vi "Module Loop.vi"(8 "error in (no error)":errorcluster, 11 "Config Alert Module in":refnum<class "Config Monitor Module.lvclass">) -> (0 "error out":errorcluster, 3 "Config Alert Module out":refnum<class "Config Monitor Module.lvclass">)   [LabVIEW 2020, in "Volatus.lvlib" / "Config Monitor Module.lvclass"]
uses:
  Config Monitor Module.lvclass
  C:/dev/lv20CE/relink/lv-volatus/Volatus/Module/Module.lvclass
  Node Config Info.ctl
  Module/Module.lvclass/Module.ctl
  MessageQ/MessageQ.lvclass/MessageQ.ctl
  Module/Module.lvclass
  Config Monitor Module.lvclass/Config Monitor Module.ctl
  ConfigMonitorInfoValue/ConfigMonitorInfoValue.lvclass/ConfigMonitorInfoValue.ctl
  Module/Parent Q.vi
  ConfigMonitorInfoValue/ConfigMonitorInfoValue.lvclass
  C:/dev/lv20CE/relink/lv-promises/Promises/Value/Value.lvclass
  <vilib>/Utility/error.llb/Error Cluster From Error Code.vi
  lv-promises/Promises/Promise/Promise.lvclass
  MessageQ/MessageQ.lvclass
panel:
  out "Config Hash":string
  out "Config Version":string
  in  "Array":T1[](array[typedef])
  # "This Node"
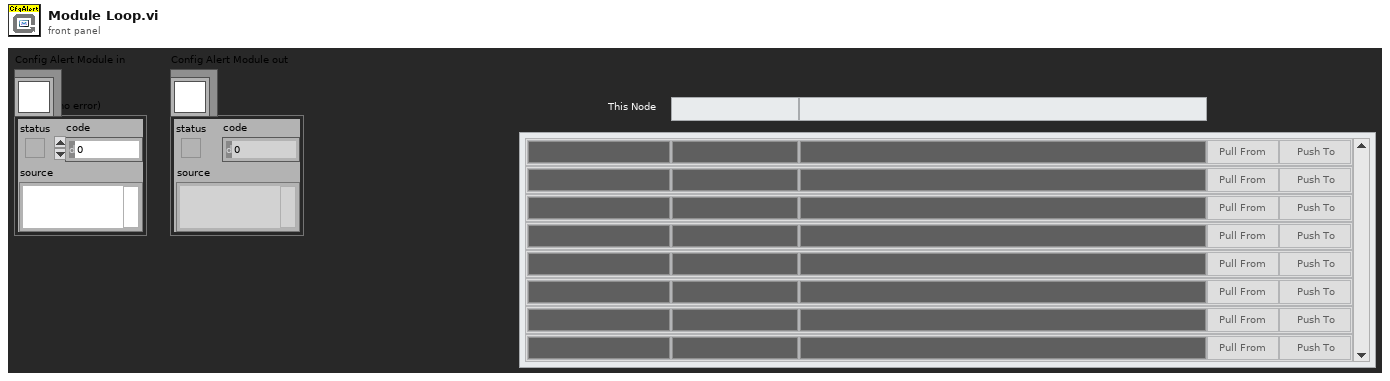
[diagram p1: front panel]
types:
  T1 = typedef "Volatus.lvlib/Config Monitor Module.lvclass/Node Config Info.ctl" = cluster{"Node":string, "Config Version":string, "Config Hash":string, "Pull":bool, "Push":bool, "Version Color":u32, "Hash Color":u32, "Node Color":u32}
  T2 = enum32{"Invalid", "Standard", "Closed", "Hidden", "Minimized", "Maximized"}
  T3 = cluster{"Node":bool, "Config Version":bool, "Config Hash":bool, "Pull":bool, "Push":bool, "Version Color":bool, "Hash Color":bool, "Node Color":bool}[]
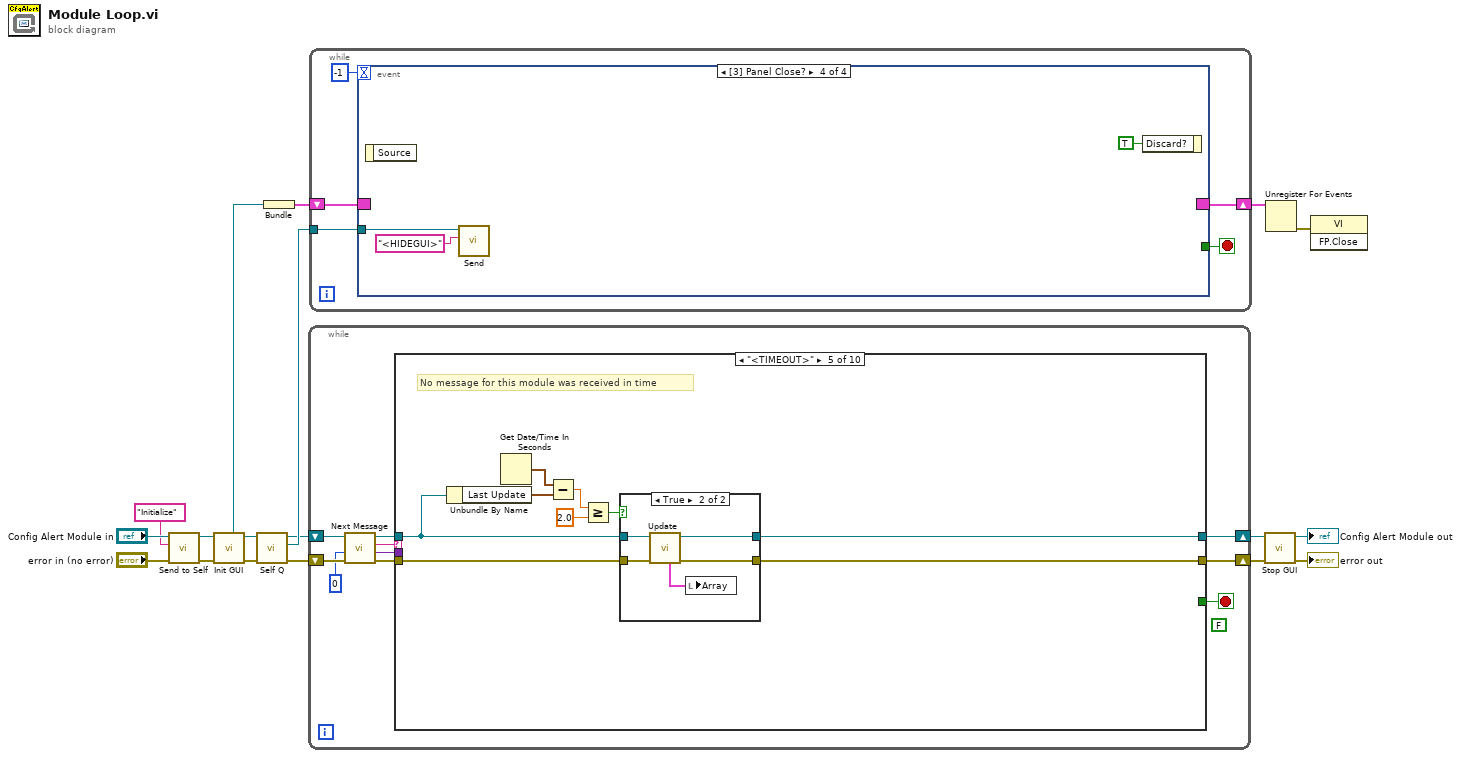
[diagram p0: block diagram]
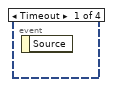
[diagram p2: hidden frame]
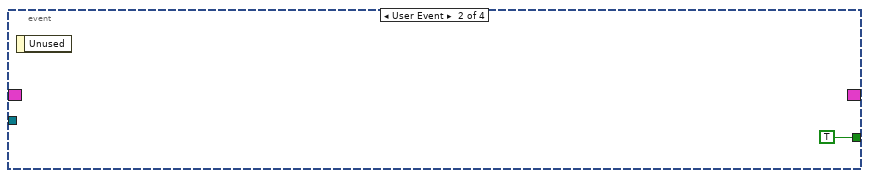
[diagram p3: hidden frame]
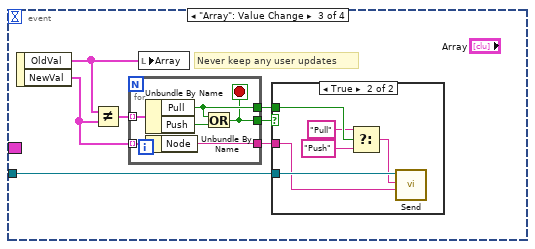
[diagram p4: hidden frame]
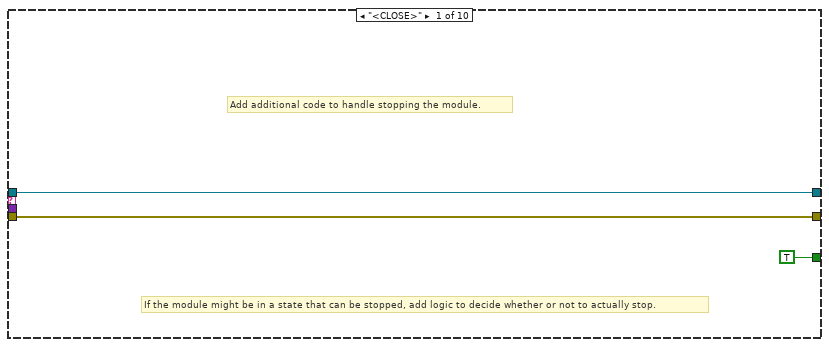
[diagram p6: hidden frame]
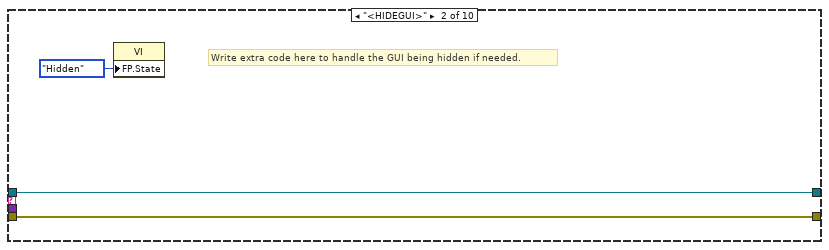
[diagram p7: hidden frame]
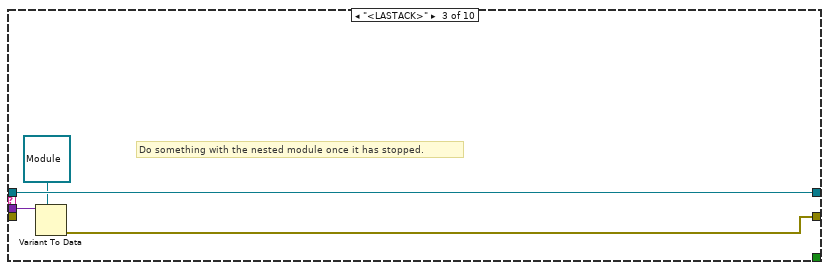
[diagram p8: hidden frame]
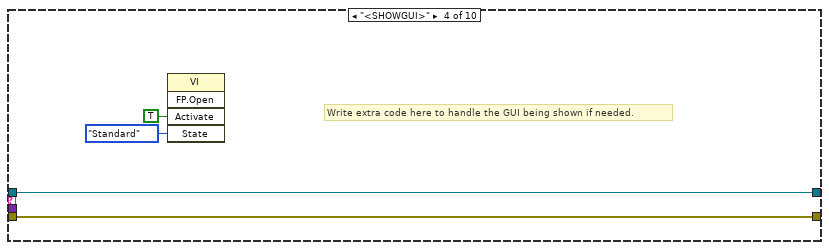
[diagram p9: hidden frame]
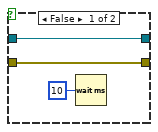
[diagram p10: hidden frame]
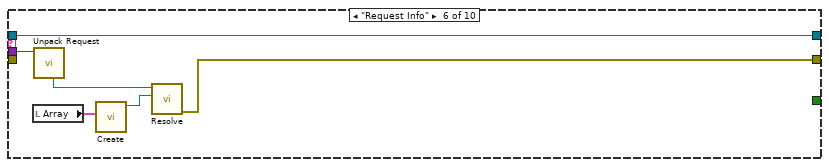
[diagram p11: hidden frame]
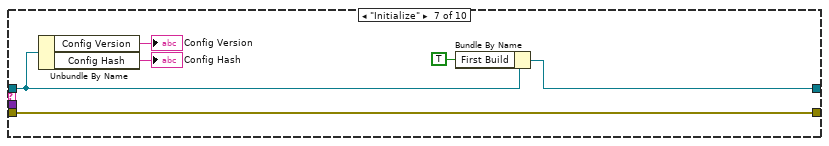
[diagram p12: hidden frame]
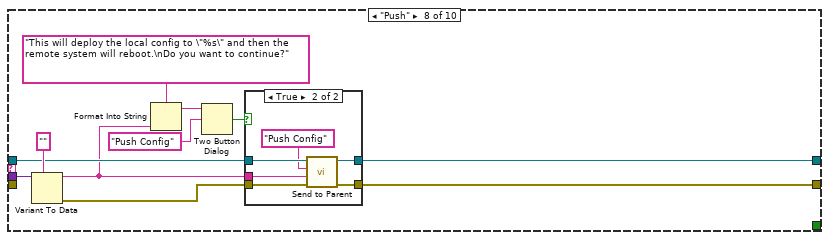
[diagram p13: hidden frame]
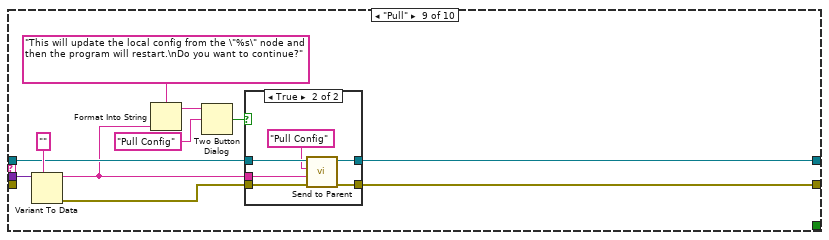
[diagram p15: hidden frame]
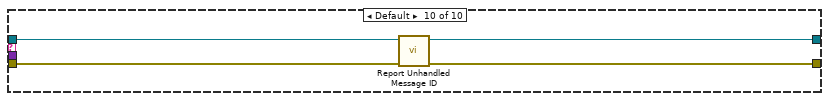
[diagram p17: hidden frame]
diagram:
  n1 = call "Send to Self.vi"("error in (no error)"="error in (no error)", "Message ID"="Initialize", "Module in"="Config Alert Module in") -> ("error out"=w4:errorcluster, "Module out"=w2:refnum<class "Config Monitor Module.lvclass">)  [unwired: 7 in]
  n2 = call "Init GUI.vi"("Module in"=w2) -> ("Module out"=w10:refnum<class "Config Monitor Module.lvclass">, "Event Reg"=w15:refnum<event-registration>)  [unwired: 9 in]
  n3 = call "Self Q.vi"("Module in"=w10) -> ("Self Q"=w9:refnum<class "MessageQ.lvclass">, "Module out"=w8:refnum<class "Config Monitor Module.lvclass">)  [unwired: 9 in]
  n4 = Bundle("Event Reg"=w15) -> (w11:cluster{"Event Reg":refnum<event-registration>})  [unwired: 1 in]
  n5 = while {
    shift-right: [w21] -> w13
    shift-left: w8 -> [w26]
    shift-right: [w20] -> w14
    shift-left: w4 -> [w25]
    stop <- w19 stop-if-true
    (unwired) FALSE
    n6 = call "Next Message.vi"("error in (no error)"=w25, "Timeout ms (-1)"=0, "Module in"=w26) -> ("error out"=w24:errorcluster, "Data"=w18:variant, "ID"=w23:string, "Module out"=w22:refnum<class "Config Monitor Module.lvclass">)  [unwired: 5 in]
    n7 = case shown="\"<TIMEOUT>\"" w23 {
      tunnel: w24 -> [w27 w31 _ w39 w49 _ w69 _ _ w111]
      tunnel: w22 -> [w28 w32 w36 w40 w46 w63 w68 w74 w93 w109]
      tunnel: [w28 w32 w36 w40 w47 w63 w65 w72 w91 w108] -> w21
      tunnel: [w27 w31 w33 w39 w48 w58 w69 w71 w90 w110] -> w20
      tunnel: [TRUE _ _ _ _ _ _ _ _ _] -> w19
      tunnel: w18 -> [_ _ w35 _ _ w62 _ w80 w99 _]
      frame "<CLOSE>" {
        # "If the module might be in a state that can be stopped, add logic to decide whether or not to actually stop."
        # "Add additional code to handle stopping the module."
      }
      frame "<HIDEGUI>" {
        # "Write extra code here to handle the GUI being hidden if needed."
        n8 = property class="VI"("FP.State"=T2."Hidden" ("Front Panel Window:State")) -> ()  [unwired: 2 in, 2 out]
      }
      frame "<LASTACK>" {
        # "Do something with the nested module once it has stopped."
        n9 = Variant To Data(type=refnum<class "Module.lvclass"> refnum ("Volatus:Module"), Variant=w35) -> (error out=w33:errorcluster)  [unwired: 1 in, 1 out]
      }
      frame "<SHOWGUI>" {
        # "Write extra code here to handle the GUI being shown if needed."
        n10 = invoke class="VI" method="FP.Open"("Activate"=TRUE ("Activate?"), "State"=T2."Standard") -> ()  [unwired: 3 in, 5 out]
      }
      frame "<TIMEOUT>" {
        # "No message for this module was received in time"
        n11 = Unbundle By Name(w46) -> ("Last Update"=w44:timestamp)
        n12 = Get Date/Time In Seconds() -> (seconds since 1Jan1904=w45:timestamp)
        n13 = Subtract(x=w45, y=w44) -> (x-y=w43:dbl)
        n14 = Greater Or Equal?(x=w43, y=2.0) -> (x >= y?=w41:bool)
        n15 = case shown="True" w41 {
          tunnel: w49 -> [w51 w57]
          tunnel: [w51 w55] -> w48
          tunnel: [w52 w54] -> w47
          tunnel: w46 -> [w52 w53]
          frame False {
            n16 = Wait (ms)(milliseconds to wait=u32 10) -> ()  [unwired: 1 out]
          }
          frame True {
            n17 = call "Update.vi"("error in (no error)"=w57, "Config Monitor Module in"=w53) -> ("error out"=w55:errorcluster, "Config Monitor Module out"=w54:refnum<class "Config Monitor Module.lvclass">, "Node Config Info"=w56:T1[])  [unwired: 7 in]
            n18 = local write "Array"(w56) -> ()
          }
        }
      }
      frame "Request Info" {
        n19 = local read "Array"() -> (w60:T1[])
        n20 = call "Unpack Request.vi"("Request Data"=w62) -> ("Promise"=w61:refnum<class "Promise.lvclass">)  [unwired: 8 in, 2 out]
        n21 = call "Create.vi"("Info"=w60) -> ("ConfigMonitorInfoValue out"=w59:refnum<class "ConfigMonitorInfoValue.lvclass">)  [unwired: 10 in]
        n22 = call "Resolve.vi"("Result"=w59, "Promise in"=w61) -> ("error out"=w58:errorcluster)  [unwired: 8 in, 1 out]
      }
      frame "Initialize" {
        n23 = Unbundle By Name(w68) -> ("Config Version"=→"Config Version":string, "Config Hash"=→"Config Hash":string)
        n24 = Bundle By Name(cluster=w68, "First Build"=TRUE) -> (w65:refnum<class "Config Monitor Module.lvclass">)
      }
      frame "Push" {
        n25 = Variant To Data(type="", Variant=w80) -> (data=w70:string, error out=w73:errorcluster)  [unwired: 1 in]
        n26 = Format Into String(format string="This will deploy the local config to \"%s\" and then the remote system will reboot.\nDo you want to continue?", w70) -> (resulting string=w77:string)  [unwired: 2 in, 1 out]
        n27 = Two Button Dialog(message=w77, 2:"Push Config" ("T button name (\"OK\")")) -> (T button?=w75:bool)  [unwired: 1 in]
        n28 = case shown="True" w75 {
          tunnel: w74 -> [w82 w88]
          tunnel: w73 -> [w81 w87]
          tunnel: [w82 w83] -> w72
          tunnel: [w81 w84] -> w71
          tunnel: w70 -> [_ w85]
          frame False {
          }
          frame True {
            n29 = call "Send to Parent.vi"("error in (no error)"=w87, "Data"=w85, "Message ID"="Push Config", "Module in"=w88) -> ("error out"=w84:errorcluster, "Module out"=w83:refnum<class "Config Monitor Module.lvclass">)  [unwired: 6 in]
          }
        }
      }
      frame "Pull" {
        n30 = Variant To Data(type="", Variant=w99) -> (data=w89:string, error out=w92:errorcluster)  [unwired: 1 in]
        n31 = Format Into String(format string="This will update the local config from the \"%s\" node and then the program will restart.\nDo you want to continue?", w89) -> (resulting string=w96:string)  [unwired: 2 in, 1 out]
        n32 = Two Button Dialog(message=w96, 2:"Pull Config" ("T button name (\"OK\")")) -> (T button?=w94:bool)  [unwired: 1 in]
        n33 = case shown="True" w94 {
          tunnel: w93 -> [w101 w107]
          tunnel: w92 -> [w100 w106]
          tunnel: [w101 w102] -> w91
          tunnel: [w100 w103] -> w90
          tunnel: w89 -> [_ w104]
          frame False {
          }
          frame True {
            n34 = call "Send to Parent.vi"("error in (no error)"=w106, "Data"=w104, "Message ID"="Pull Config", "Module in"=w107) -> ("error out"=w103:errorcluster, "Module out"=w102:refnum<class "Config Monitor Module.lvclass">)  [unwired: 6 in]
          }
        }
      }
      frame Default {
        n35 = call "Report Unhandled Message ID.vi"("error in (no error)"=w111, "Module in"=w109) -> ("error out"=w110:errorcluster, "Module out"=w108:refnum<class "Config Monitor Module.lvclass">)  [unwired: 8 in]
      }
    }
  }
  n36 = while {
    tunnel: w9 -> [w116]
    shift-right: [w114] -> w12
    shift-left: w11 -> [w115]
    stop <- w113 stop-if-true
    n37 = event shown="[3] Panel Close?" {
      selector: w115 -> [_ _ _ _]
      dyn-events: [_ _ _ _] -> w114
      timeout: -1 -> [_ _ _ _]
      tunnel: w116 -> [_ _ w120 w138]
      tunnel: [_ TRUE _ _] -> w113
      event Timeout {
        n38 = event-data() -> ()  [unwired: 1 in, 1 out]
      }
      event User Event {
        n39 = event-data() -> ()  [unwired: 1 in, 1 out]
      }
      event "Array": Value Change {
        # "Never keep any user updates"
        n40 = event-data() -> ("OldVal"=w124:T1[], "NewVal"=w122:T1[])  [unwired: 1 in]
        n41 = Not Equal?(x=w124, y=w122) -> (x != y?=w123:T3)
        n42 = for {
          tunnel: w123 -> [w136] mode=indexing
          tunnel: w122 -> [w135] mode=indexing
          tunnel: [w133] -> w121
          tunnel: [w134] -> w118
          tunnel: [w131] -> w119
          stop <- w131 stop-if-true
          n43 = Unbundle By Name(w136) -> ("Pull"=w133:bool, "Push"=w132:bool)
          n44 = Unbundle By Name(w135) -> ("Node"=w134:string)
          n45 = Or(x=w133, y=w132) -> (x .or. y?=w131:bool)
        }
        n46 = local write "Array"(w124) -> ()
        n47 = case shown="True" w119 {
          tunnel: w121 -> [_ w130]
          tunnel: w120 -> [_ w127]
          tunnel: w118 -> [_ w125]
          frame False {
          }
          frame True {
            n48 = Select(t="Pull", s=w130, f="Push") -> (s? t:f=w126:string)
            n49 = call "Send.vi"("Data"=w125, "ID"=w126, "MessageQ in"=w127) -> ()  [unwired: 7 in, 2 out]
          }
        }
      }
      event Panel Close? {
        n50 = event-data() -> ()  [unwired: 1 in, 1 out]
        n51 = call "Send.vi"("ID"="<HIDEGUI>", "MessageQ in"=w138) -> ()  [unwired: 8 in, 2 out]
        n52 = event-data("Discard?"=TRUE) -> ()  [unwired: 1 in, 1 out]
      }
    }
  }
  n53 = call "Stop GUI.vi"("error in (no error)"=w14, "Module in"=w13) -> ("error out"=→"error out":errorcluster, "Module out"=→"Config Alert Module out":refnum<class "Config Monitor Module.lvclass">)  [unwired: 8 in]
  n54 = Unregister For Events(event registration refnum=w12) -> (error out=w16:errorcluster)  [unwired: 1 in]
  n55 = invoke class="VI" method="FP.Close"(error in=w16) -> ()  [unwired: 2 in, 3 out]
